vi "Database.Handler-Kill.vi"(8 "error in":errorcluster) -> (0 "error out":errorcluster)   [LabVIEW 2016]
uses:
  Database.Handler.Action.ctl
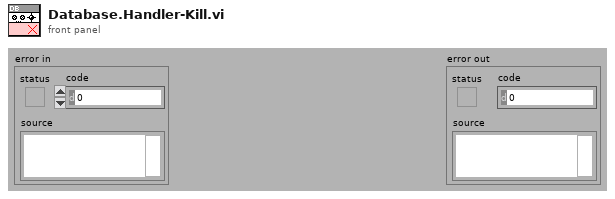
[diagram p1: front panel]
types:
  T1 = typedef "Database.Handler.Action.ctl" = enum32{"idle", "constructor", "destructor", "--- DB.Handler ---", "Setup", "Reconnect", "ReconnectAll", "ReconnectOne", "ExportData"}
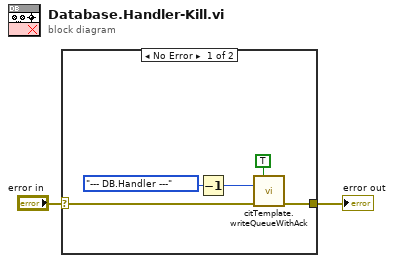
[diagram p0: block diagram]
diagram:
  n1 = case shown="No Error" "error in" {
    selector: "error in" -> [w5 w8]
    tunnel: [w7 w8] -> w1
    frame No Error {
      n2 = Decrement(x=Database.Handler.Action."--- DB.Handler ---" ("Action")) -> (x-1=w4:T1)
      n3 = call "citTemplate.writeQueueWithAck.vi"("High priority (F)"=TRUE, "event in"=w4, "error in (no error)"=w5) -> ("error out"=w7:errorcluster)  [unwired: 10 in, 2 out]
    }
    frame Error {
    }
  }
  "error out" <- w1
